vi "Update Extra ADAM Chs.vi"(2 "Extra Ch Values":string[](array[string]), 3 "Extra Ch Names":string[](array[string])) -> ()   [LabVIEW 2022 SP3]
uses:
  Globals/Meas_global.vi
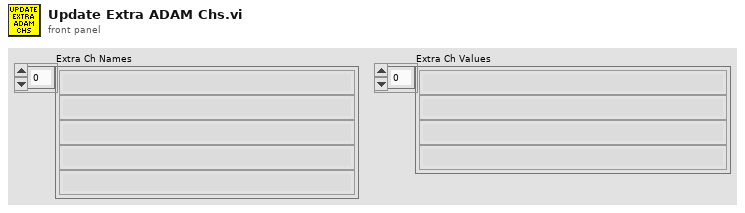
[diagram p1: front panel]
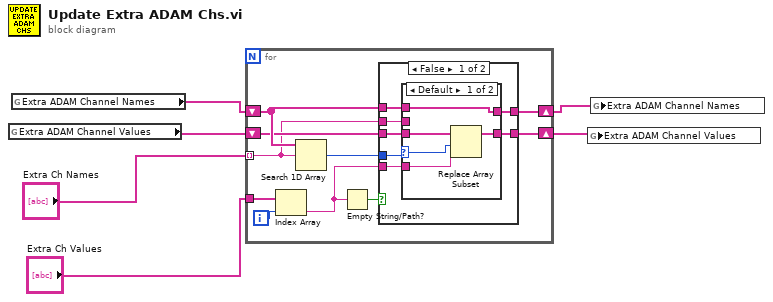
[diagram p0: block diagram]
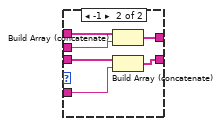
[diagram p2: hidden frame]
diagram:
  n1 = global read "Meas_global.vi" "Extra ADAM Channel Values"() -> (w1:string[])
  n2 = global read "Meas_global.vi" "Extra ADAM Channel Names"() -> (w2:string[])
  n3 = for {
    tunnel: "Extra Ch Names" -> [w11] mode=indexing
    shift-right: [w15] -> w4
    shift-left: w2 -> [w14]
    shift-right: [w12] -> w3
    shift-left: w1 -> [w13]
    tunnel: "Extra Ch Values" -> [w9]
    i -> [w8]
    n4 = Index Array(array=w9, index=w8) -> (element=w7:string)
    n5 = Search 1D Array(1D array=w14, element=w11) -> (index of element=w16:i32)  [unwired: 1 in]
    n6 = Empty String/Path?(string/path=w7) -> (empty?=w10:bool)
    n7 = case shown="False" w10 {
      tunnel: w16 -> [w23 _]
      tunnel: [w22 w36] -> w15
      tunnel: w14 -> [w21 w36]
      tunnel: w13 -> [w20 w35]
      tunnel: [w19 w35] -> w12
      tunnel: w11 -> [w18 _]
      tunnel: w7 -> [w17 _]
      frame False {
        n8 = case shown="Default" w23 {
          selector: w23 -> [w25 _]
          tunnel: w21 -> [w28 w34]
          tunnel: [w28 w33] -> w22
          tunnel: w18 -> [_ w32]
          tunnel: w17 -> [w24 w31]
          tunnel: w20 -> [w27 w30]
          tunnel: [w26 w29] -> w19
          frame Default {
            n9 = Replace Array Subset(array=w27, new element=w24, index=w25) -> (w26:string[])
          }
          frame -1 {
            n10 = Build Array (concatenate)(w34, w32) -> (w33:string[])
            n11 = Build Array (concatenate)(w30, w31) -> (w29:string[])
          }
        }
      }
      frame True {
      }
    }
  }
  n12 = global write "Meas_global.vi" "Extra ADAM Channel Values"(w3) -> ()
  n13 = global write "Meas_global.vi" "Extra ADAM Channel Names"(w4) -> ()
